vi "ABS_Motor.vi"(9 "Boolean":bool, 11 "Numeric":dbl) -> (3 "Numeric 2":dbl)   [LabVIEW 2016]
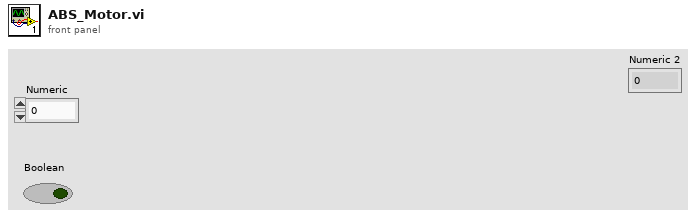
[diagram p1: front panel]
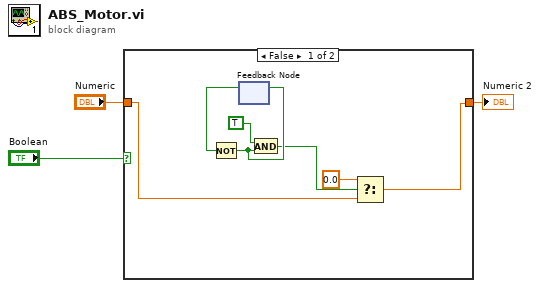
[diagram p0: block diagram]
diagram:
  n1 = case shown="False" "Boolean" {
    tunnel: "Numeric" -> [w8 w11]
    tunnel: [w7 w11] -> w2
    frame False {
      n2 = feedback #1() -> (w6:bool)  [unwired: 1 in]
      n3 = Not(x=w6) -> (.not. x?=w5:bool)
      n4 = feedback-in #1(w5) -> ()
      n5 = And(x=TRUE, y=w5) -> (x .and. y?=w4:bool)
      n6 = Select(t=0.0, s=w4, f=w8) -> (s? t:f=w7:dbl)
    }
    frame True {
    }
  }
  "Numeric 2" <- w2
